vi "Get Service Class Instances.vi"() -> (3 "service instances":refnum<class "ServiceBase.lvclass">[](array[class]))   [LabVIEW 2021, in "Stream_server.lvlib"]
uses:
  Stream_server.lvlib
  <vilib>/gRPC/LabVIEW gRPC Servicer/ServiceBase/ServiceBase.lvclass
  RPC Service/Random_Data/Random_Data.lvclass
  C:/Program Files/National Instruments/LabVIEW 2021/vi.lib/gRPC/LabVIEW gRPC Servicer/ServiceBase/ServiceBase.lvclass
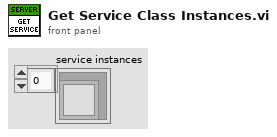
[diagram p1: front panel]
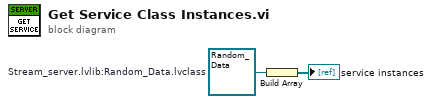
[diagram p0: block diagram]
diagram:
  w1 = refnum<class "Random_Data.lvclass"> refnum  # Stream_server.lvlib:Random_Data.lvclass
  n1 = Build Array(w1) -> (→"service instances":refnum<class "Random_Data.lvclass">[])
